vi "Arm Motors.vi"() -> ()   [LabVIEW 2018]
uses:
  <vilib>/Rock Robotics/WPI/ThirdParty/Phoenix-LabVIEW/Motor Controller/Controls/CTRE_Phoenix_MotorControl_NeutralMode.ctl
  <vilib>/Rock Robotics/WPI/ThirdParty/Phoenix-LabVIEW/Motor Controller/Controls/CTRE_Phoenix_MotorControl_ControlMode.ctl
  Framework/Robot Global Data.vi
  <vilib>/ptbypt/NI_PtbyPt.lvlib
panel:
  in  "Drop-Off Angle":dbl=110.0
  in  "Pick-Up Angle":dbl=110.0
  out "Waveform Chart":T1(graph)
  in  "Proportional Slowdown":dbl=40.0
  in  "Min speed":dbl=0.06 min=0.0 max=1.0 step=0.01
  out "Arm Angle Error":dbl format="%.2f"
  in  "Motor Tuning":T2={"Max Motor Speed"=1.0, "Decel Angle (Deg)"=40.0, "Deadband Angle (Deg)"=0.5} {"Max Motor Speed" min=0.0 max=1.0 step=0.05}
  in  "Loop Time":u32=20
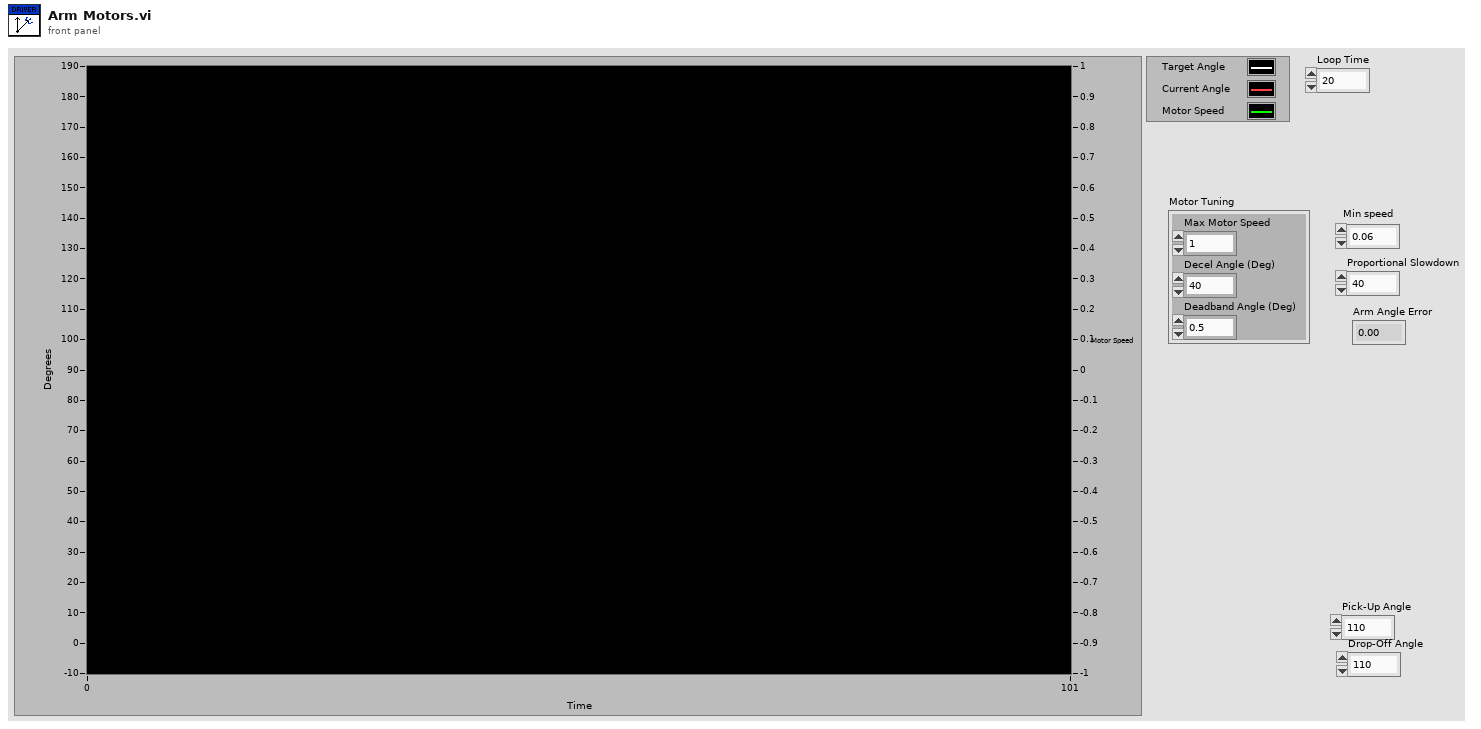
[diagram p1: front panel]
types:
  T1 = cluster{"Target Angle":dbl, "Current Angle":dbl, "Motor Speed":dbl}[]
  T2 = cluster{"Max Motor Speed":dbl, "Decel Angle (Deg)":dbl, "Deadband Angle (Deg)":dbl}
  T3 = typedef "CTRE_Phoenix_MotorControl_NeutralMode.ctl" = enum8{"EEPROMSetting", "Override to Coast", "Override to Brake"}
  T4 = typedef "WPI_MotorControlDeviceRef.ctl" = cluster{"DeviceStatus":errorcluster, "Type":T5, "PWM":cluster{"PWM Channel":T6, "DeadBand":T7}, "CAN":cluster{"Device Number":u8, "SetOutput VI Ref":variant, "GetOutput VI Ref":variant, "Enable VI Ref":variant, "Disable VI Ref":variant, "Data":variant}, "Invert":bool, "DIO PWM":cluster{"PWM \"Enable\" Channel":T6, "DIOChannel":T8, "PWM Rate":dbl}}
  T5 = typedef "WPI_MotorControlType.ctl" = enum16{"PWM", "CAN", "DIO PWM"}
  T6 = typedef "FPGA_DIOPWMChannel.ctl" = enum8{"PWM 0", "PWM 1", "PWM 2", "PWM 3", "PWM 4", "PWM 5", "PWM 6", "PWM 7", "PWM 8", "PWM 9", "PWM MXP 0", "PWM MXP 1", "PWM MXP 2", "PWM MXP 3", "PWM MXP 4", "PWM MXP 5", "PWM MXP 6", "PWM MXP 7", "PWM MXP 8", "PWM MXP 9", "Invalid"}
  T7 = typedef "WPI_PWMDeadband.ctl" = cluster{"Name":string, "maxPositivePwm":i32, "minPositivePwm":i32, "centerPwm":i32, "maxNegativePwm":i32, "minNegativePwm":i32, "angularRange":u16}
  T8 = typedef "FPGA_DIOChannel.ctl" = enum8{"DIO 0", "DIO 1", "DIO 2", "DIO 3", "DIO 4", "DIO 5", "DIO 6", "DIO 7", "DIO 8", "DIO 9", "DIO MXP 0", "DIO MXP 1", "DIO MXP 2", "DIO MXP 3", "DIO MXP 4", "DIO MXP 5", "DIO MXP 6", "DIO MXP 7", "DIO MXP 8", "DIO MXP 9", "DIO MXP 10", "DIO MXP 11", "DIO MXP 12", "DIO MXP 13", "DIO MXP 14", "DIO MXP 15", "SPI Port CS1", "SPI Port CS2", "SPI Port CS3", "SPI Port MISO", "SPI Port MOSI", "Invalid"}
  T9 = cluster{"Target Angle":dbl, "Current Angle":dbl, "Motor Speed":dbl}
  T10 = typedef "WPI_DriverStationRobotMode2.ctl" = enum16{"Autonomous Disabled", "Autonomous Enabled", "Teleop Disabled", "Teleop Enabled", "Disconnected", "Finish", "Test Disabled", "Test Enabled", "Emergency Stopped"}
  T11 = typedef "CTRE_Phoenix_MotorControl_ControlMode.ctl" = u16
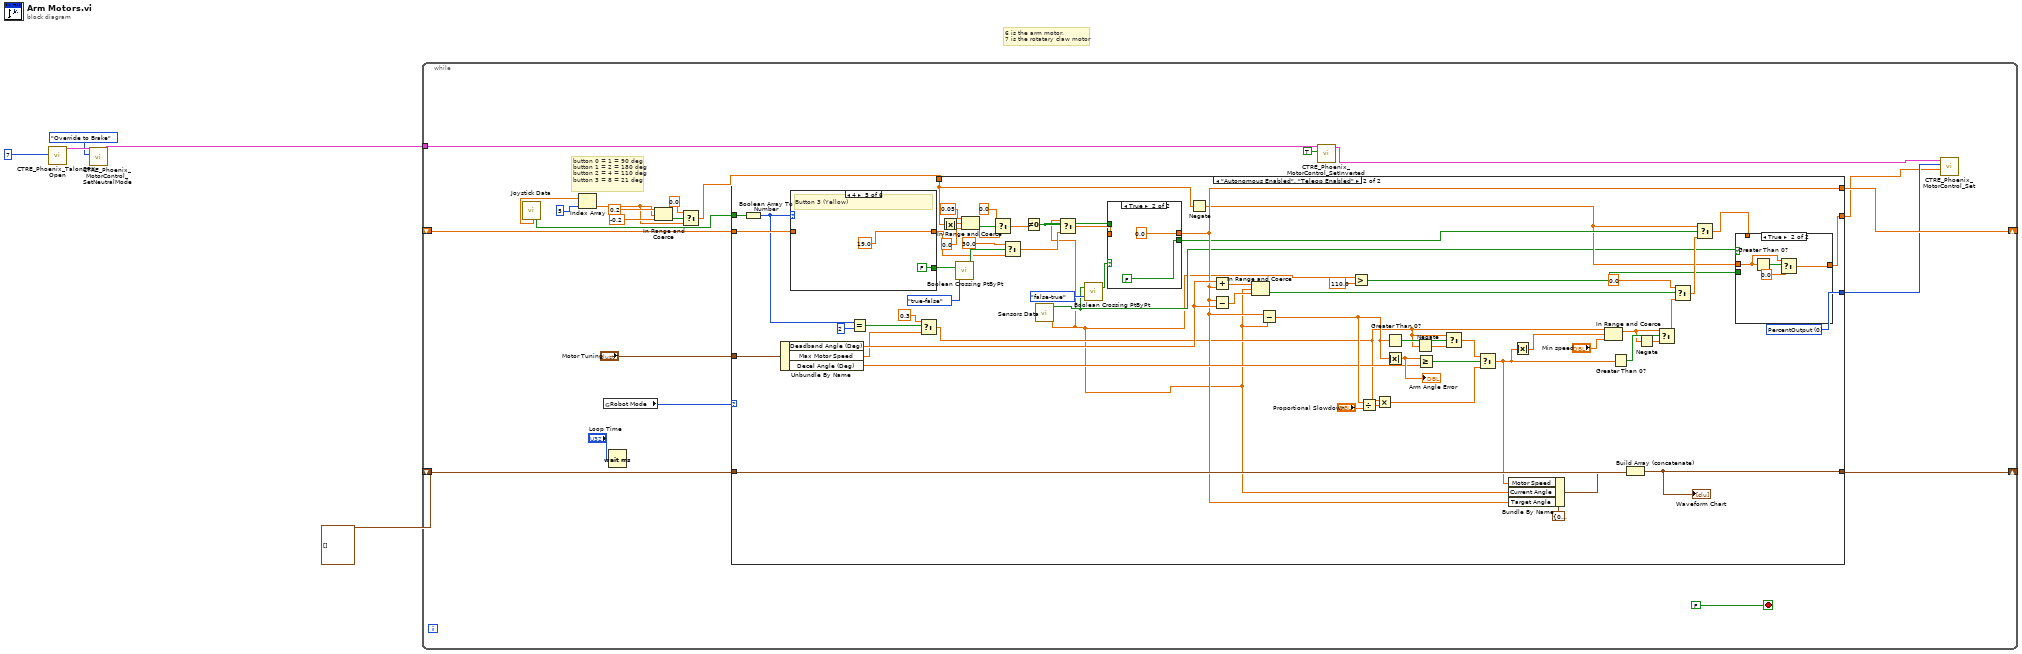
[diagram p0: block diagram]
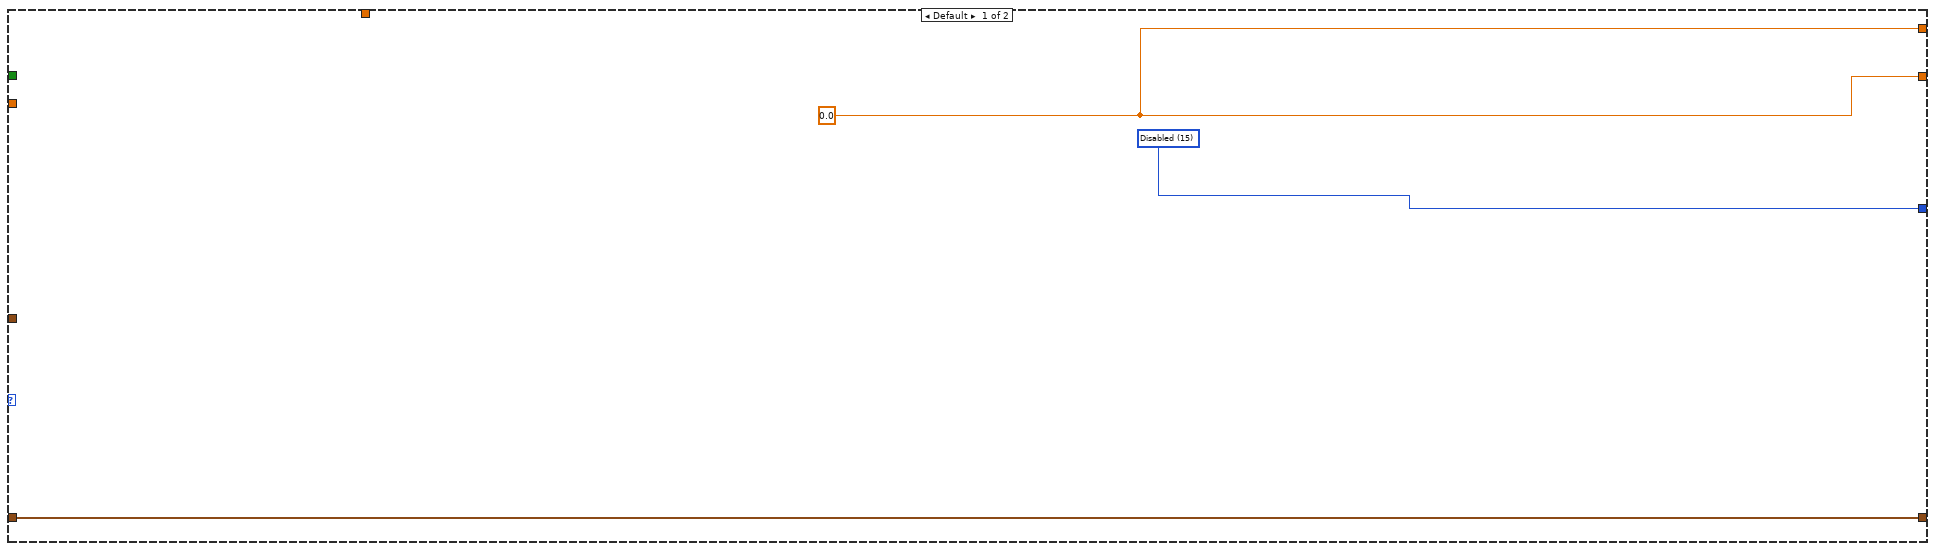
[diagram p2: hidden frame]
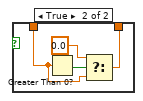
[diagram p4: hidden frame]
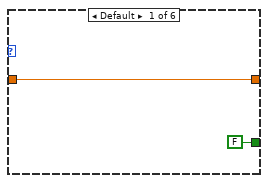
[diagram p6: hidden frame]
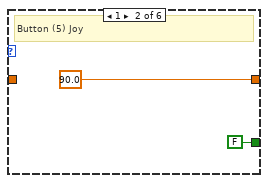
[diagram p7: hidden frame]
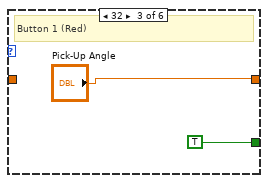
[diagram p8: hidden frame]
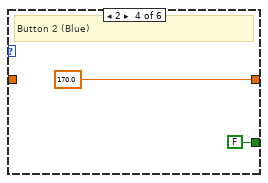
[diagram p9: hidden frame]
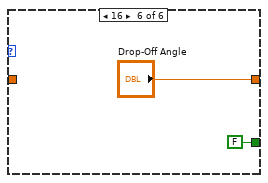
[diagram p10: hidden frame]
diagram:
  # "6 is the arm motor, \n7 is the rotatary claw motor"
  n1 = call <vilib>:"CTRE_Phoenix_TalonSRX_Open.vi"("Device Number"=7) -> ("CAN Talon SRX Ref"=w4:T4)  [unwired: 9 in, 1 out]
  n2 = call <vilib>:"CTRE_Phoenix_MotorControl_SetNeutralMode.vi"("Motor Control Neutral Mode"=CTRE_Phoenix_MotorControl_NeutralMode."Override to Brake", "PhoenixMotorControlDevRef"=w4) -> ("PhoenixMotorControlDevRef"=w1:T4)  [unwired: 8 in, 1 out]
  n3 = while {
    tunnel: w1 -> [w20]
    shift-right: [w23] -> _
    shift-left: T1 [] -> [w24]
    shift-right: [w19] -> _
    shift-left: _ -> [w18]
    stop <- FALSE stop-if-true
    # "button 0 = 1 = 90 deg\nbutton 1 = 2 = 180 deg\nbutton 2 = 4 = 110 deg\nbutton 3 = 8 = 21 deg"
    n4 = call "Joystick Data.vi"() -> ("Xbox 360 Joy Out"=w7:dbl[], "Xbox 360 Out"=w6:bool[])  [unwired: 12 in, 6 out]
    n5 = Index Array(array=w7, index=5) -> (element=w8:dbl)
    n6 = global read "Robot Global Data.vi" "Robot Mode"() -> (w27:T10)
    n7 = Wait (ms)(milliseconds to wait="Loop Time") -> ()  [unwired: 1 out]
    n8 = In Range and Coerce(upper limit=0.2, x=w8, lower limit=-0.2) -> (In Range?=w11:bool)  [unwired: 1 out]
    n9 = Select(t=0.0, s=w11, f=w8) -> (s? t:f=w12:dbl)
    n10 = case shown="\"Autonomous Enabled\", \"Teleop Enabled\"" w27 {
      tunnel: [w30 w81] -> w17
      tunnel: [w28 w43] -> w15
      tunnel: w24 -> [w29 w85]
      tunnel: [w29 w83] -> w23
      tunnel: "Motor Tuning" -> [_ w61]
      tunnel: w6 -> [_ w70]
      tunnel: [w28 w62] -> w19
      tunnel: w18 -> [_ w68]
      tunnel: w12 -> [_ w51]
      frame Default {
        w30 = T11 15 items=["PercentOutput"=0, "Position"=1, "Velocity"=2, "Current"=3, "Follower"=5, "MotionProfile"=6, "MotionMagic"=7, "MotionProfileArc"=10, "Disabled"=15] ("Control Mode")
        w28 = 0.0 ("f")
      }
      frame "Autonomous Enabled", "Teleop Enabled" {
        w81 = T11 0 items=["PercentOutput"=0, "Position"=1, "Velocity"=2, "Current"=3, "Follower"=5, "MotionProfile"=6, "MotionMagic"=7, "MotionProfileArc"=10, "Disabled"=15] ("Control Mode")
        n11 = Boolean Array To Number(Boolean array=w70) -> (number=w55:u32)
        n12 = Unbundle By Name(w61) -> ("Deadband Angle (Deg)"=w69:dbl, "Max Motor Speed"=w56:dbl, "Decel Angle (Deg)"=w82:dbl)
        n13 = case shown="4" w55 {
          tunnel: [w112 90.0 ("index") "Pick-Up Angle" 170.0 ("index") 19.0 ("index") "Drop-Off Angle"] -> w38
          tunnel: w68 -> [w112 _ _ _ _ _]
          tunnel: [FALSE FALSE TRUE FALSE FALSE FALSE] -> w41
          frame Default {
          }
          frame 1 {
            # "Button (5) Joy"
          }
          frame 32 {
            # "Button 1 (Red)"
          }
          frame 2 {
            # "Button 2 (Blue)"
          }
          frame 4 {
            # "Button 3 (Yellow)"
          }
          frame 16 {
          }
        }
        n14 = Equal?(x=w55, y=u32 2) -> (x = y?=w59:bool)
        n15 = Select(t=0.3, s=w59, f=w56) -> (s? t:f=w58:dbl)
        n16 = Absolute Value(x=w51) -> (abs(x)=w50:dbl)
        n17 = call <vilib>:"Boolean Crossing PtByPt.vi"("direction"=enum16{"either", "false-true", "true-false"}."true-false", "input"=w41) -> ("crossing"=w39:bool)  [unwired: 1 in]
        n18 = In Range and Coerce(upper limit=0.05, x=w50, lower limit=0.0) -> (coerced(x)=w46:dbl, In Range?=w47:bool)
        n19 = Select(t=0.0, s=w47, f=w46) -> (s? t:f=w44:dbl)
        n20 = Select(t=30.0, s=w39, f=w38) -> (s? t:f=w36:dbl)
        n21 = Not Equal To 0?(x=w44) -> (x != 0?=w52:bool)
        n22 = call "Sensors Data.vi"() -> ("Distance Out"=w33:dbl, "Limit Up Out"=w34:bool)  [unwired: 8 in, 2 out]
        n23 = Select(t=w33, s=w52, f=w36) -> (s? t:f=w64:dbl)
        n24 = call <vilib>:"Boolean Crossing PtByPt.vi"("direction"=enum16{"either", "false-true", "true-false"}."false-true", "input"=w34) -> ("crossing"=w65:bool)  [unwired: 1 in]
        n25 = case shown="True" w65 {
          tunnel: w64 -> [w108 _]
          tunnel: [w108 0.0 ("t")] -> w62
          tunnel: [w107 FALSE ("Manual Target")] -> w54
          tunnel: w52 -> [w107 _]
          frame False {
          }
          frame True {
          }
        }
        n26 = Negate(x=w51) -> (-x=w42:dbl)
        n27 = Add(x=w69, y=w62) -> (x+y=w94:dbl)
        n28 = Subtract(x=w62, y=w69) -> (x-y=w93:dbl)
        n29 = In Range and Coerce(upper limit=w94, x=w33, lower limit=w93) -> (In Range?=w71:bool)  [unwired: 1 out]
        n30 = Subtract(x=w62, y=w33) -> (x-y=w87:dbl)
        n31 = Greater?(x=w33, y=110.0) -> (0:w31:bool)
        n32 = Divide(x=w87, y="Proportional Slowdown") -> (x/y=w67:dbl)
        n33 = Multiply(x=w58, y=w67) -> (x*y=w77:dbl)
        n34 = Greater Than 0?(x=w87) -> (x > 0?=w89:bool)
        n35 = Absolute Value(x=w87) -> (abs(x)=w92:dbl)
        "Arm Angle Error" <- w92
        n36 = Negate(x=w58) -> (-x=w88:dbl)
        n37 = Greater Or Equal?(x=w92, y=w82) -> (x >= y?=w91:bool)
        n38 = Select(t=w58, s=w89, f=w88) -> (s? t:f=w90:dbl)
        n39 = Select(t=w90, s=w91, f=w77) -> (s? t:f=w63:dbl)
        n40 = Bundle By Name(cluster=T9 {"Target Angle"=0.0, "Current Angle"=0.0, "Motor Speed"=0.0}, "Motor Speed"=w63, "Current Angle"=w33, "Target Angle"=w62) -> (w84:T9)
        n41 = Absolute Value(x=w63) -> (abs(x)=w76:dbl)
        n42 = In Range and Coerce(upper limit=w58, x=w76, lower limit="Min speed") -> (coerced(x)=w74:dbl)  [unwired: 1 out]
        n43 = Greater Than 0?(x=w63) -> (x > 0?=w75:bool)
        n44 = Build Array (concatenate)(w85, w84) -> (w83:T1)
        "Waveform Chart" <- w83
        n45 = Negate(x=w74) -> (-x=w73:dbl)
        n46 = Select(t=w74, s=w75, f=w73) -> (s? t:f=w72:dbl)
        n47 = Select(t=0.0, s=w71, f=w72) -> (s? t:f=w53:dbl)
        n48 = Select(t=w42, s=w54, f=w53) -> (s? t:f=w35:dbl)
        n49 = case shown="True" w34 {
          tunnel: w42 -> [_ w103]
          tunnel: [w95 w105] -> w43
          tunnel: w35 -> [w96 _]
          tunnel: w31 -> [w97 _]
          frame False {
            n50 = case shown="False" w97 {
              tunnel: w96 -> [w98 w100]
              tunnel: [w98 w99] -> w95
              frame False {
              }
              frame True {
                n51 = Greater Than 0?(x=w100) -> (x > 0?=w102:bool)
                n52 = Select(t=0.0, s=w102, f=w100) -> (s? t:f=w99:dbl)
              }
            }
          }
          frame True {
            n53 = Greater Than 0?(x=w103) -> (x > 0?=w104:bool)
            n54 = Select(t=w103, s=w104, f=0.0) -> (s? t:f=w105:dbl)
          }
        }
      }
    }
    n55 = call <vilib>:"CTRE_Phoenix_MotorControl_SetInverted.vi"("Invert?"=TRUE, "PhoenixMotorControlDevRef"=w20) -> ("PhoenixMotorControlDevRef"=w16:T4)  [unwired: 8 in, 1 out]
    n56 = call <vilib>:"CTRE_Phoenix_MotorControl_Set.vi"("Output"=w15, "Control Mode"=w17, "PhoenixMotorControlDevRef"=w16) -> ()  [unwired: 7 in, 2 out]
  }
